vi "Watchport Comm.vi"(5 "Close session":bool=TRUE, 7 "Initialization":bool=TRUE, 8 "error in":errorcluster, 10 "Watchport command":string="TF", 11 "Watchport COM #":refnum<visa-resource-name>="COM3") -> (0 "error out":errorcluster, 1 "value":sgl, 2 "watchport reply":string, 3 "COM port out":refnum<visa-resource-name>="COM3", 4 "return count":u32)   [LabVIEW 2018]
uses:
  <vilib>/Instr/_visa.llb/VISA Configure Serial Port (Instr).vi
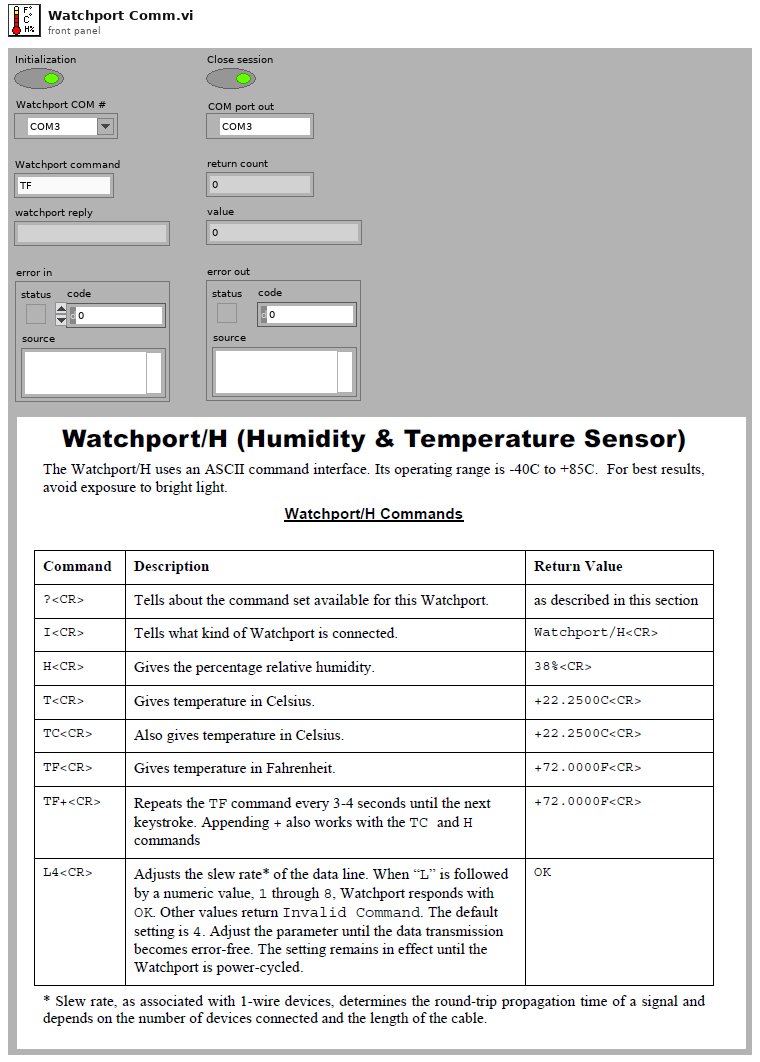
[diagram p1: front panel]
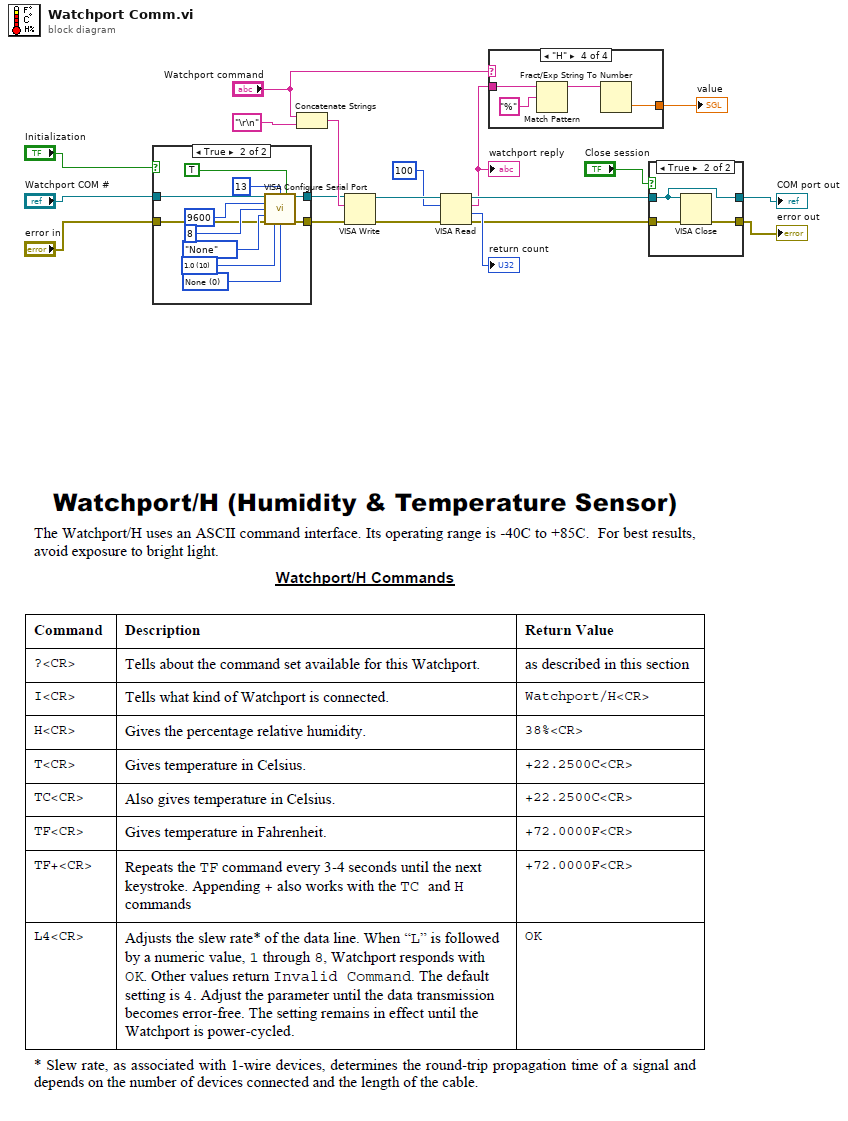
[diagram p0: block diagram]
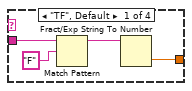
[diagram p2: hidden frame]
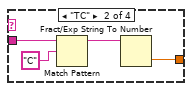
[diagram p3: hidden frame]
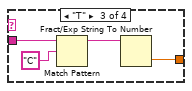
[diagram p4: hidden frame]
diagram:
  n1 = case shown="True" "Initialization" {
    tunnel: [w21 w22] -> w13
    tunnel: [w20 w26] -> w11
    tunnel: "Watchport COM #" -> [w21 w25]
    tunnel: "error in" -> [w20 w24]
    frame False {
    }
    frame True {
      w31 = u16 0 items=["None", "XON/XOFF", "RTS/CTS", "XON/XOFF & RTS/CTS", "DTR/DSR", "XON/XOFF & DTR/DSR"] ("flow control (0:none)")
      w30 = u16 10 items=["1.0"=10, "1.5"=15, "2.0"=20] ("stop bits (10: 1 bit)")
      n2 = call-poly "VISA Configure Serial Port"("VISA resource name"=w25, "termination char\n(0xA = '\\n' = LF)"=u8 13 ("termination char\n(0xA = '\\n' = LF)"), "Enable Termination\nChar (T)"=TRUE ("Enable Termination\nChar (T)"), "baud rate (9600)"=u32 9600, "data bits (8)"=u16 8, "parity (0:none)"=enum16{"None", "Odd", "Even", "Mark", "Space"}."None", "error in (no error)"=w24, "stop bits (10: 1 bit)"=w30, "flow control (0:none)"=w31) -> ("VISA resource name out"=w22:refnum<visa-resource-name>, "error out"=w26:errorcluster)  [unwired: 5 out]
    }
  }
  n3 = Concatenate Strings("Watchport command", "\r\n" ("write buffer")) -> (w18:string)
  n4 = VISA Write(VISA resource name=w13, write buffer=w18, error in (no error)=w11) -> (VISA resource name out=w16:refnum<visa-resource-name>, error out=w17:errorcluster)  [unwired: 1 out]
  n5 = VISA Read(VISA resource name=w16, byte count=u32 100, error in (no error)=w17) -> (VISA resource name out=w5:refnum<visa-resource-name>, read buffer=w3:string, return count=→"return count":u32, error out=w4:errorcluster)
  "watchport reply" <- w3
  n6 = case shown="\"H\"" "Watchport command" {
    tunnel: w3 -> [w36 w37 w41 w46]
    tunnel: [w33 w38 w42 w45] -> w2
    frame "TF", Default {
      n7 = Match Pattern(string=w36, regular expression="F") -> (before substring=w34:string)  [unwired: 1 in, 3 out]
      n8 = Fract/Exp String To Number(string=w34) -> (number=w33:dbl)  [unwired: 4 out]
    }
    frame "TC" {
      n9 = Match Pattern(string=w37, regular expression="C") -> (before substring=w39:string)  [unwired: 1 in, 3 out]
      n10 = Fract/Exp String To Number(string=w39) -> (number=w38:dbl)  [unwired: 4 out]
    }
    frame "T" {
      n11 = Match Pattern(string=w41, regular expression="C") -> (before substring=w43:string)  [unwired: 1 in, 3 out]
      n12 = Fract/Exp String To Number(string=w43) -> (number=w42:dbl)  [unwired: 4 out]
    }
    frame "H" {
      n13 = Match Pattern(string=w46, regular expression="%") -> (before substring=w47:string)  [unwired: 1 in, 3 out]
      n14 = Fract/Exp String To Number(string=w47) -> (number=w45:dbl)  [unwired: 4 out]
    }
  }
  "value" <- w2
  n15 = case shown="True" "Close session" {
    tunnel: w5 -> [w50 w53]
    tunnel: w4 -> [w49 w52]
    tunnel: [w50 w53] -> w7
    tunnel: [w49 w51] -> w8
    frame False {
    }
    frame True {
      n16 = VISA Close(VISA resource name=w53, error in (no error)=w52) -> (error out=w51:errorcluster)
    }
  }
  "COM port out" <- w7
  "error out" <- w8
